vi "FrameCmdB.vi"(6 "idx":u16, 7 "data":u32, 8 "error in":errorcluster, 9 "DataType":enum8{"Int", " float"}(ring), 10 "CommType":enum8{"Set", "Get"}(ring), 11 "cmd_id":u16) -> (0 "error out":errorcluster, 2 "output array":u8[](array[numeric]))   [LabVIEW 2017]
uses:
  Crc16DLL.dll
panel:
  out "CRCout":u16 format="%.0x"
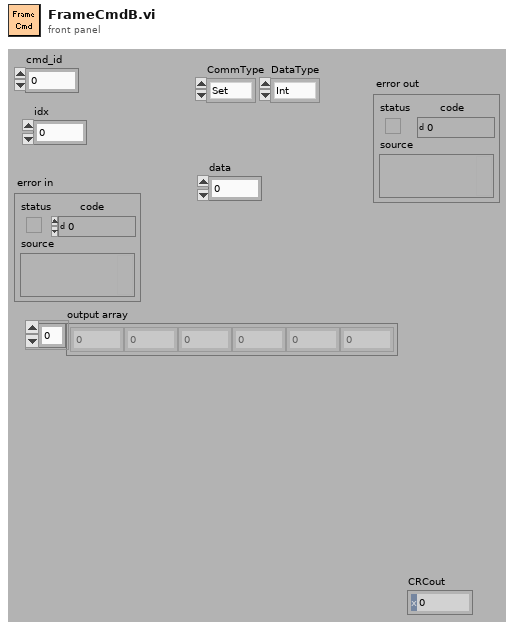
[diagram p1: front panel]
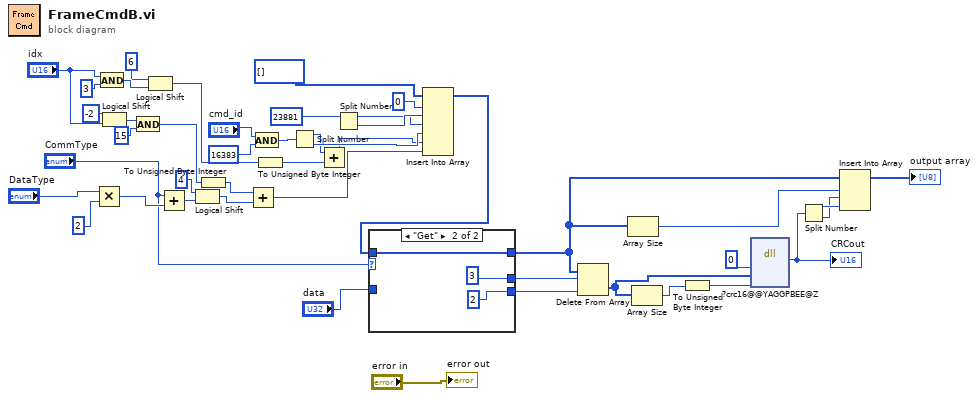
[diagram p0: block diagram]
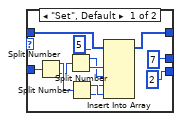
[diagram p2: hidden frame]
diagram:
  n1 = Multiply(x="DataType", y=u8 2) -> (x*y=w36:u8)
  n2 = And(x="idx", y=u16 3) -> (x .and. y?=w10:u16)
  n3 = Logical Shift(y=i16 -2, x="idx") -> (x << y=w20:u16)
  n4 = And(x=w20, y=u16 15) -> (x .and. y?=w17:u16)
  n5 = Logical Shift(y=i16 6, x=w10) -> (x << y=w9:u16)
  n6 = Add(x="CommType", y=w36) -> (x+y=w25:u8)
  n7 = Logical Shift(y=i8 4, x=w25) -> (x << y=w18:u8)
  n8 = To Unsigned Byte Integer(number=w17) -> (unsigned 8bit integer=w15:u8)
  n9 = Add(x=w15, y=w18) -> (x+y=w16:u8)
  n10 = And(x="cmd_id", y=u16 16383) -> (x .and. y?=w14:u16)
  n11 = To Unsigned Byte Integer(number=w9) -> (unsigned 8bit integer=w11:u8)
  n12 = Split Number(x=w14) -> (hi(x)=w13:u8, lo(x)=w39:u8)
  n13 = Add(x=w13, y=w11) -> (x+y=w12:u8)
  n14 = Split Number(x=u16 23881 ("MagicNumber")) -> (hi(x)=w41:u8, lo(x)=w42:u8)
  n15 = Insert Into Array(array=u8[] [] ("array_in"), index=0, new element #1=w42, new element #2=w41, new element #3=w39, new element #4=w12, new element #5=w16) -> (w5:u8[])
  n16 = case shown="\"Get\"" "CommType" {
    tunnel: w5 -> [w57 w60]
    tunnel: [w56 w60] -> w4
    tunnel: [7 ("length") 3 ("length")] -> w3
    tunnel: [2 ("index") 2 ("index")] -> w2
    tunnel: "data" -> [w51 _]
    frame "Set", Default {
      n17 = Split Number(x=w51) -> (hi(x)=w53:u16, lo(x)=w52:u16)
      n18 = Split Number(x=w52) -> (hi(x)=w49:u8, lo(x)=w50:u8)
      n19 = Split Number(x=w53) -> (hi(x)=w48:u8, lo(x)=w47:u8)
      n20 = Insert Into Array(array=w57, index=5, new element #1=w50, new element #2=w49, new element #3=w47, new element #4=w48) -> (w56:u8[])
    }
    frame "Get" {
    }
  }
  n21 = Delete From Array(array=w4, length=w3, index=w2) -> (deleted portion=w28:u8[])  [unwired: 1 out]
  n22 = Array Size(array=w4) -> (size(s)=w30:i32)
  n23 = Array Size(array=w28) -> (size(s)=w29:i32)
  n24 = To Unsigned Byte Integer(number=w29) -> (unsigned 8bit integer=w35:u8)
  n25 = dll-call lib="C:/Projects/Marvin CAN UTD/MarvinATP/Crc16DLL.dll" fn="?crc16@@YAGGPBEE@Z"("CRC"=u16 0, "buffer"=w28, "len"=w35) -> ("return type"=w33:u16)  [unwired: 6 in, 2 out]
  "CRCout" <- w33
  n26 = Split Number(x=w33) -> (hi(x)=w32:u8, lo(x)=w31:u8)
  n27 = Insert Into Array(array=w4, index=w30, new element #1=w31, new element #2=w32) -> (→"output array":u8[])
  "error out" <- "error in"
